vi "Count edges simple.vi"() -> ()   [LabVIEW 2020]
uses:
  <vilib>/Utility/error.llb/DialogType.ctl
  <vilib>/DAQmx/read.llb/DAQmx Read (Counter U32 1Chan 1Samp).vi
  <vilib>/DAQmx/create/channels.llb/DAQmx Create Channel (CI-Count Edges).vi
  <vilib>/DAQmx/miscellaneous.llb/DAQmx Fill In Error Info.vi
  <resource>/objmgr/daqmx.rc
panel:
  in  "Active Edge":i32(ring)=10280 items=["Rising"=10280, "Falling"=10171]
  in  "Input Terminal":tag="/Dev1/PFI0"
  in  "Counter":tag="Dev1/ctr0"
  in  "Trigger Type":T1(tab)=enum."Digital Pause"
  in  "Edge":i32(ring)=10280 items=["Rising"=10280, "Falling"=10171]
  in  "Digital Trigger Source":tag
  in  "Pause When":i32(ring)=10214 items=["High"=10192, "Low"=10214]
  in  "Pause Trigger Source":tag="/Dev1/PFI9"
  in  "Count Reset Terminal":tag
  in  "Edge 2":i32(ring)=10280 items=["Rising"=10280, "Falling"=10171]
  in  "Stop":bool
  in  "Loop Time (ms)":u32=1000
  out "Count":u32=1624984
  out "Current count":u32
  # "To configure and use a trigger or the count reset you must have the necessary tab selected above.  Not all hardware supports the above options--refer to your device documentation for more info."
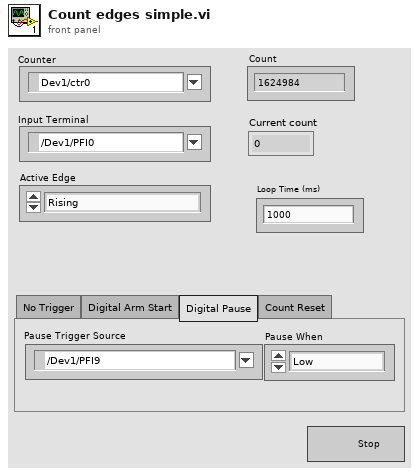
[diagram p1: front panel]
types:
  T1 = enum32{"No Trigger", "Digital Arm Start", "Digital Pause", "Count Reset"}
  T2 = typedef "DialogType.ctl" = u16
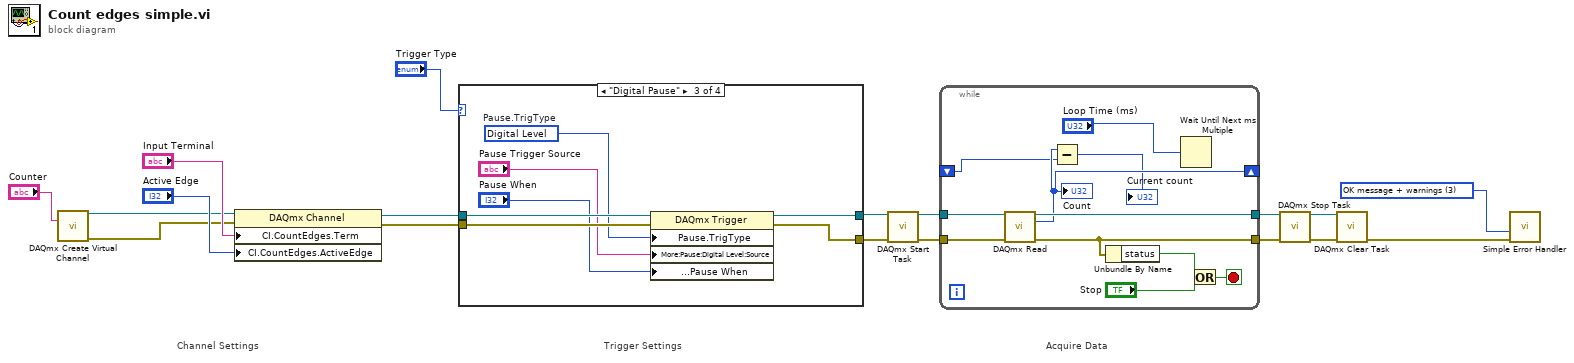
[diagram p0: block diagram]
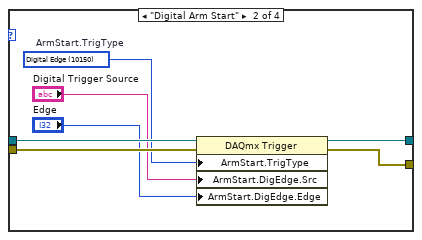
[diagram p3: hidden frame]
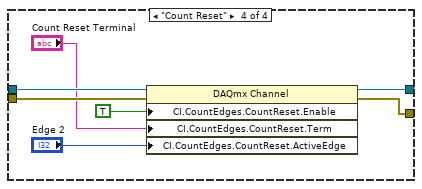
[diagram p4: hidden frame]
diagram:
  w1 = T2 3 items=["no dialog", "OK message", "continue or stop message", "OK message + warnings", "continue/stop + warnings"] ("type of dialog (OK msg:1)")
  # "Acquire Data"
  # "Trigger Settings"
  # "Channel Settings"
  n1 = call-poly <vilib>:"DAQmx Create Virtual Channel.vi"("counter"="Counter") -> ("task out"=w9:refnum<k21>, "error out"=w8:errorcluster)  [unwired: 13 in]
  n2 = property class="DAQmx Channel"(reference=w9, error in=w8, "CI.CountEdges.Term"="Input Terminal", "CI.CountEdges.ActiveEdge"="Active Edge") -> (reference out=w6:refnum<k21>, error out=w7:errorcluster)
  n3 = case shown="\"Digital Pause\"" "Trigger Type" {
    tunnel: w6 -> [w20 w27 w34 w41]
    tunnel: w7 -> [w19 w24 w31 w38]
    tunnel: [w20 w26 w33 w40] -> w16
    tunnel: [w19 w25 w32 w39] -> w15
    frame "No Trigger", Default {
    }
    frame "Digital Arm Start" {
      w21 = 10150 items=["Digital Edge"=10150, "None"=10230]  # ArmStart.TrigType
      n4 = property class="DAQmx Trigger"(reference=w27, error in=w24, "ArmStart.TrigType"=w21, "ArmStart.DigEdge.Src"="Digital Trigger Source", "ArmStart.DigEdge.Edge"="Edge") -> (reference out=w26:refnum<k21>, error out=w25:errorcluster)
    }
    frame "Digital Pause" {
      w30 = 10152 items=["Analog Level"=10101, "Analog Window"=10103, "Digital Level"=10152, "Digital Pattern"=10398, "None"=10230]  # Pause.TrigType
      n5 = property class="DAQmx Trigger"(reference=w34, error in=w31, "Pause.TrigType"=w30, "More:Pause:Digital Level:Source"="Pause Trigger Source", "More:Pause:Digital Level:Pause When"="Pause When") -> (reference out=w33:refnum<k21>, error out=w32:errorcluster)
    }
    frame "Count Reset" {
      n6 = property class="DAQmx Channel"(reference=w41, error in=w38, "CI.CountEdges.CountReset.Enable"=TRUE, "CI.CountEdges.CountReset.Term"="Count Reset Terminal", "CI.CountEdges.CountReset.ActiveEdge"="Edge 2") -> (reference out=w40:refnum<k21>, error out=w39:errorcluster)
    }
  }
  n7 = call <vilib>:"DAQmx Start Task.vi"("task/channels in"=w16, "error in"=w15) -> ("task out"=w14:refnum<k21>, "error out"=w13:errorcluster)  [unwired: 12 in]
  n8 = while {
    tunnel: w14 -> [w52]
    tunnel: w13 -> [w51]
    tunnel: [w48] -> w4
    tunnel: [w49] -> w5
    shift-right: [w45] -> _
    shift-left: _ -> [w44]
    stop <- w50 stop-if-true
    n9 = call-poly <vilib>:"DAQmx Read.vi"("task/channels in"=w52, "error in"=w51) -> ("task out"=w49:refnum<k21>, "data"=w45:u32, "error out"=w48:errorcluster)  [unwired: 11 in]
    "Count" <- w45
    n10 = Subtract(x=w45, y=w44) -> (x-y=→"Current count":u32)
    n11 = Unbundle By Name(w48) -> ("status"=w47:bool)
    n12 = Wait Until Next ms Multiple(millisecond multiple="Loop Time (ms)") -> ()  [unwired: 1 out]
    n13 = Or(x=w47, y="Stop") -> (x .or. y?=w50:bool)
  }
  n14 = call <vilib>:"DAQmx Stop Task.vi"("task/channels in"=w5, "error in"=w4) -> ("task out"=w2:refnum<k21>, "error out"=w3:errorcluster)  [unwired: 12 in]
  n15 = call <vilib>:"DAQmx Clear Task.vi"("task in"=w2, "error in"=w3) -> ("error out"=w12:errorcluster)  [unwired: 13 in]
  n16 = call <vilib>:"Simple Error Handler.vi"("type of dialog (OK msg:1)"=w1, "error in (no error)"=w12) -> ()  [unwired: 3 in, 5 out]
